vi "Send Ping.vi"(8 "error in (no error)":errorcluster, 11 "WebSocket Connection in":refnum<class "WebSocket Connection.lvclass">) -> (0 "error out":errorcluster, 3 "WebSocket Connection out":refnum<class "WebSocket Connection.lvclass">)   [LabVIEW 2021, in "WebSocket Actors.lvlib" / "WebSocket Connection.lvclass"]
doc: "Sends a Ping packet to the peer. Used by the \"Keepalive Hearbeat\" actor within the Keepalive mechanism"
uses:
  WebSocket Connection.lvclass
  WebSocket Connection.lvclass/WebSocket Connection.ctl
  <vilib>/GPower/Error/Library/SplitAppended.vi
  <vilib>/GPower/Error/Library/AppendErrors.vi
  <vilib>/GPower/Error/Library/Append/AppendMulti.vi
  <vilib>/GPower/Error/Library/SubVIs/ExplanationToError.vi
  <vilib>/dlg_ctls.llb/Space Constant.vi
  <vilib>/Utility/error.llb/Trim Whitespace.vi
  <vilib>/Utility/error.llb/Error Code Database.vi
  <vilib>/GPower/Error/Library/Append/AppendSingle.vi
  <vilib>/GPower/Error/GPError.lvlib
  <vilib>/LS Instruments AG/LV-WebSockets/LV WebSockets.lvlib
panel:
  in  "timeout ms (5000)":i32=5000
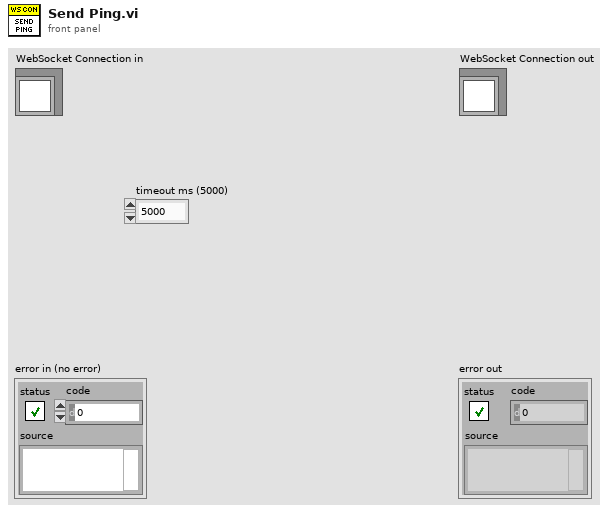
[diagram p1: front panel]
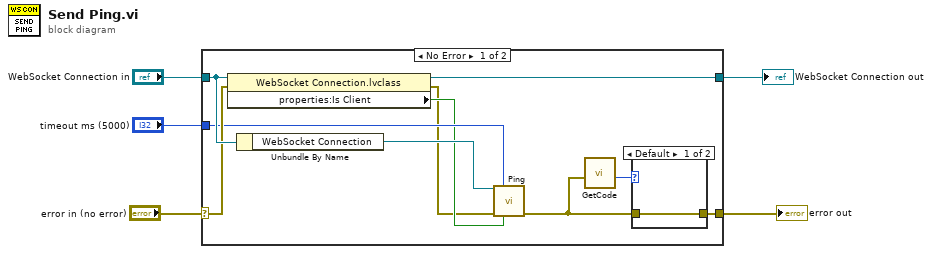
[diagram p0: block diagram]
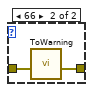
[diagram p2: hidden frame]
diagram:
  n1 = case shown="No Error" "error in (no error)" {
    selector: "error in (no error)" -> [w13 w20]
    tunnel: [w11 w20] -> w3
    tunnel: [w14 w19] -> w2
    tunnel: "WebSocket Connection in" -> [w15 w19]
    tunnel: "timeout ms (5000)" -> [w10 _]
    frame No Error {
      n2 = property class="WebSocket Connection.lvclass"(reference=w15, error in=w13) -> (reference out=w14:refnum<class "WebSocket Connection.lvclass">, error out=w7:errorcluster, "properties:Is Client"=w8:bool)
      n3 = Unbundle By Name(w15) -> ("WebSocket Connection"=w9:refnum<k5>)
      n4 = call <vilib>:"Ping.vi"("WebSocket Connection in"=w9, "timeout ms (5000)"=w10, "error in (no error)"=w7, "Mask payload?"=w8) -> ("error out"=w6:errorcluster)  [unwired: 10 in, 1 out]
      n5 = call <vilib>:"GetCode.vi"("Error in"=w6) -> ("Code"=w12:i32)  [unwired: 10 in]
      n6 = case shown="Default" w12 {
        tunnel: [w16 w17] -> w11
        tunnel: w6 -> [w16 w18]
        frame Default {
        }
        frame 66 {
          n7 = call <vilib>:"ToWarning.vi"("Error in"=w18) -> ("Warning out"=w17:errorcluster)  [unwired: 10 in]
        }
      }
    }
    frame Error {
    }
  }
  "error out" <- w3
  "WebSocket Connection out" <- w2
